vi "SetOutputPortNo.vi"(8 "error in (no error)":errorcluster, 10 "#ports":u8=1 min=1 max=8, 11 "DIO64Output.lvclass in":refnum<class "DIO64Output.lvclass">) -> (0 "error out":errorcluster, 3 "DIO64Output.lvclass out":refnum<class "DIO64Output.lvclass">)   [LabVIEW 2009, in "Hardware.lvlib" / "Channels.lvlib" / "DIO64Output.lvclass"]
uses:
  DIO64Output.lvclass
  DIO64Output.lvclass/DIO64Output.ctl
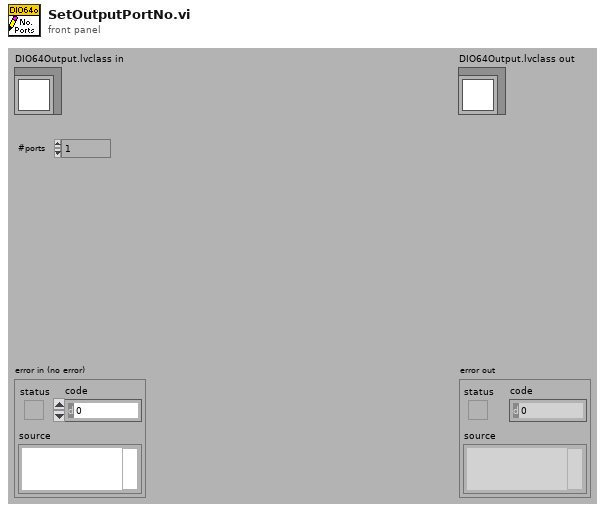
[diagram p1: front panel]
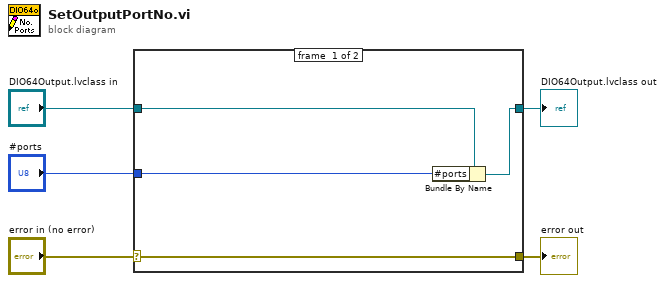
[diagram p0: block diagram]
diagram:
  n1 = case shown="No Error" "error in (no error)" {
    selector: "error in (no error)" -> [w9 w10]
    tunnel: [w9 w10] -> w4
    tunnel: [w7 w11] -> w2
    tunnel: "DIO64Output.lvclass in" -> [w8 w11]
    tunnel: "#ports" -> [w6 _]
    frame #0 {
      n2 = Bundle By Name(cluster=w8, "#ports"=w6) -> (w7:refnum<class "DIO64Output.lvclass">)
    }
    frame #1 {
    }
  }
  "error out" <- w4
  "DIO64Output.lvclass out" <- w2
